vi "Wire Non-Nodes to Nodes.vi"(7 "What to Wire":T1, 8 "error in (no error)":errorcluster, 10 "Nodes":refnum<vi>[](array[refnum]), 11 "Available Non-Nodes in":T2[](array[typedef])) -> (0 "error out":errorcluster, 2 "Any Changes?":bool, 3 "Available Non-Nodes out":T2[](array[typedef]))   [LabVIEW 2016]
uses:
  <resource>/dialog/QuickDrop/plugins/_WireMultipleSupport/Available Non-Node.ctl
  <resource>/dialog/QuickDrop/plugins/_WireMultipleSupport/What to Wire.ctl
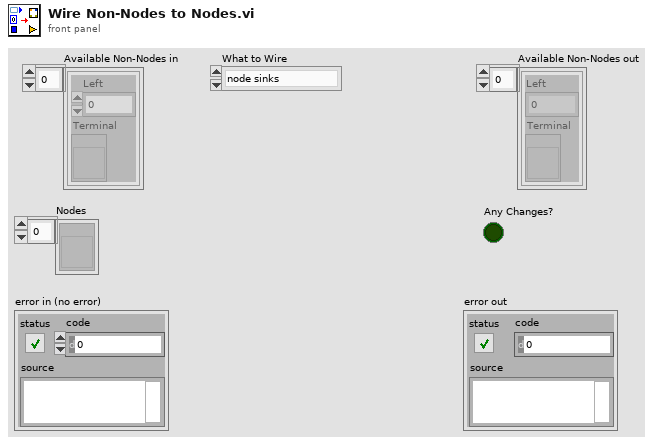
[diagram p1: front panel]
types:
  T1 = typedef "What to Wire.ctl" = enum16{"node sinks", "node sources"}
  T2 = typedef "Available Non-Node.ctl" = cluster{"Left":i32, "Terminal":refnum<vi>}
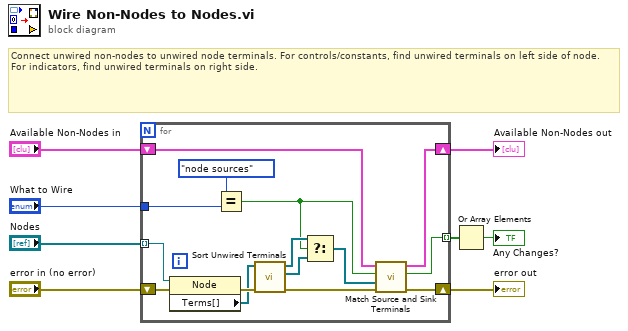
[diagram p0: block diagram]
diagram:
  # "Connect unwired non-nodes to unwired node terminals. For controls/constants, find unwired terminals on left side of node. For indicators, find unwired terminals on right side."
  n1 = for {
    shift-right: [w18] -> w5
    shift-left: "error in (no error)" -> [w23]
    tunnel: "Nodes" -> [w22] mode=indexing
    shift-right: [w20] -> w7
    shift-left: "Available Non-Nodes in" -> [w21]
    tunnel: [w19] -> w3 mode=indexing
    tunnel: "What to Wire" -> [w14]
    n2 = property class="Node"(reference=w22, error in=w23) -> (error out=w17:errorcluster, "Terms[]"=w15:refnum<vi>[])  [unwired: 1 out]
    n3 = Equal?(x=What_to_Wire."node sources", y=w14) -> (x = y?=w9:bool)
    n4 = call <resource>:"Sort Unwired Terminals.vi"("error in (no error)"=w17, "Terms in"=w15) -> ("error out"=w16:errorcluster, "Unwired Sink Terms"=w11:refnum<vi>[], "Unwired Source Terms"=w12:refnum<vi>[])  [unwired: 7 in]
    n5 = Select(t=w12, s=w9, f=w11) -> (s? t:f=w10:refnum<vi>[])
    n6 = call <resource>:"Match Source and Sink Terminals.vi"("error in (no error)"=w16, "Node Terminals"=w10, "Node Sources?"=w9, "Available Non-Nodes in"=w21) -> ("error out"=w18:errorcluster, "Any Changes?"=w19:bool, "Available Non-Nodes out"=w20:T2[])  [unwired: 5 in]
  }
  "Available Non-Nodes out" <- w7
  "error out" <- w5
  n7 = Or Array Elements(Boolean array=w3) -> (logical OR=→"Any Changes?":bool)
